vi "U32 Endianness Swap.vi"(8 "MSB":u8, 9 "2":u8, 10 "1":u8, 11 "LSB":u8) -> (2 "Out":u32)   [LabVIEW 2015]
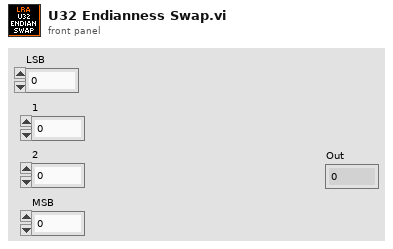
[diagram p1: front panel]
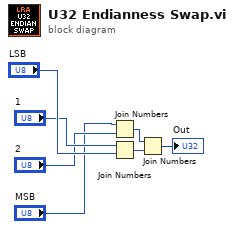
[diagram p0: block diagram]
diagram:
  n1 = Join Numbers(hi="MSB", lo="2") -> ((hi.lo)=w7:u16)
  n2 = Join Numbers(hi="1", lo="LSB") -> ((hi.lo)=w6:u16)
  n3 = Join Numbers(hi=w7, lo=w6) -> ((hi.lo)=→"Out":u32)
